vi "Autotune.vi"() -> ()   [LabVIEW 2018]
uses:
  <vilib>/Utility/file.llb/Read Delimited Spreadsheet (DBL).vi
  <vilib>/Utility/file.llb/Read Delimited Spreadsheet (string).vi
panel:
  out "Freq":dbl
  out "Note":string
  in  "NotesPath":path
  in  "FreqsPath":path
  in  "NormalizedFreq":dbl
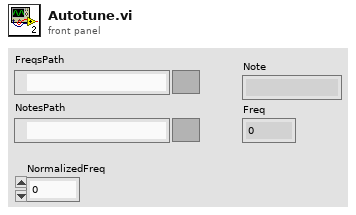
[diagram p1: front panel]
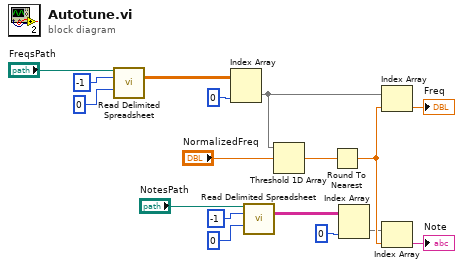
[diagram p0: block diagram]
diagram:
  n1 = call-poly <vilib>:"Read Delimited Spreadsheet.vi"("file path (dialog if empty)"="FreqsPath", "number of rows (all:-1)"=-1, "max characters/row  (no limit:0)"=0) -> ("all rows"=w14:dbl[][])  [unwired: 7 in, 5 out]
  n2 = Index Array(array=w14, index (col)=0 ("index (row)")) -> (element=w5:dbl[])  [unwired: 1 in]
  n3 = call-poly <vilib>:"Read Delimited Spreadsheet.vi"("file path (dialog if empty)"="NotesPath", "number of rows (all:-1)"=-1, "max characters/row  (no limit:0)"=0) -> ("all rows"=w9:string[][])  [unwired: 7 in, 5 out]
  n4 = Threshold 1D Array(2:"NormalizedFreq", 3:w5) -> (0:w6:dbl)  [unwired: 1 in]
  n5 = Round To Nearest(number=w6) -> (nearest integer value=w4:dbl)
  n6 = Index Array(array=w9, index (col)=0 ("index (row)")) -> (element=w3:string[])  [unwired: 1 in]
  n7 = Index Array(array=w5, index=w4) -> (element=→"Freq":dbl)
  n8 = Index Array(array=w3, index=w4) -> (element=→"Note":string)
